vi "Set RX Output Divider.vi"(8 "error in":errorcluster, 10 "rx output divider":T1, 11 "eye scan in":refnum<class "niHighSpeedSerial Eye Scan v1 Host.lvclass">) -> (0 "error out":errorcluster, 3 "eye scan out":refnum<class "niHighSpeedSerial Eye Scan v1 Host.lvclass">)   [LabVIEW 2014, in "niHighSpeedSerial Eye Scan v1 Host.lvclass"]
doc: "Sets the RX Output Divider. This must match the values configured with RXRATE and RXOUT_DIV.\n\n<B>Input Parameters</B>\n\n<B>error in</B> describes error conditions that occur before this node runs. This input provides standard 'error in' functionality.\n\n<B>rx output divider</B> represents the configuration of the receiver output divider. This should match the values configured with RXRATE and RXOUT_DIV.\nenum values: 1,2,4,8,16\n\n<B>eye scan in</B> Takes in a reference to your session from the previous VI.\n\n<B>Output Parameters</B>\n\n<B>error out</B> contains error information. This output provides standard 'error out' functionality.\n\n<B>eye scan out</B> passes a reference to your session to the next VI."
uses:
  <instrlib>/niHighSpeedSerial/Eye Scan/v1/Host/Eye Scan/niHighSpeedSerial Eye Scan v1 Host.lvclass
  <instrlib>/niHighSpeedSerial/Eye Scan/v1/Host/Common/Public/RX Output Divider.ctl
  <instrlib>/niHighSpeedSerial/Eye Scan/v1/Host/Eye Scan/niHighSpeedSerial Eye Scan v1 Host.lvclass/niHighSpeedSerial Eye Scan v1 Host.ctl
  <vilib>/Utility/error.llb/Error Cluster From Error Code.vi
  <vilib>/ErrorRing/Error Ring.xnode
  <instrlib>/niHighSpeedSerial/Eye Scan/v1/Host/Common/niHighSpeedSerial Eye Scan Common v1 Host.lvlib
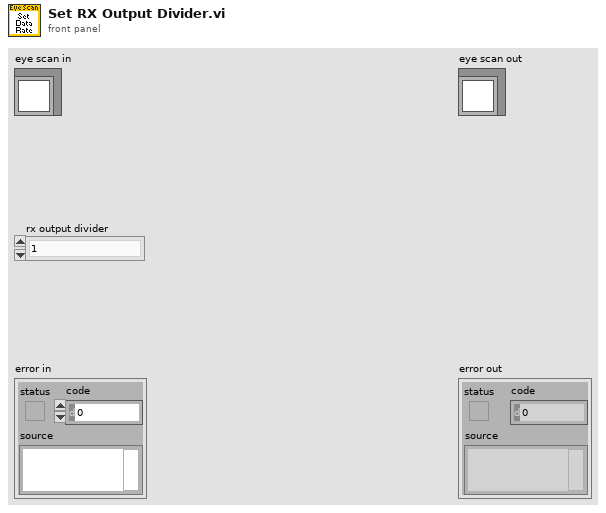
[diagram p1: front panel]
types:
  T1 = typedef "niHighSpeedSerial Eye Scan Common v1 Host.lvlib/RX Output Divider.ctl" = enum16{"1", "2", "4", "8", "16"}
  T2 = typedef "niHighSpeedSerial Eye Scan v1 Host.lvclass/Private Data.ctl" = cluster{"instruction target":refnum<class "niInstr Instruction Target v1 Host.lvclass">, "channels":T3[], "measure state":T4, "rx output divider":T1, "equalization mode":T5, "rx data width":T6, "BER floor":dbl, "number of points completed":i32, "rx output divider configured?":bool, "equalization mode configured?":bool, "rx data width configured?":bool}
  T3 = typedef "niHighSpeedSerial Eye Scan v1 Host.lvclass/Channel Data.ctl" = cluster{"instance":u8, "channel":refnum<class "niHighSpeedSerial Eye Scan Single Point v1 Host.lvclass">, "point iterator":refnum<class "niHighSpeedSerial Eye Scan Point Iterator v1 Host.lvclass">}
  T4 = typedef "niHighSpeedSerial Eye Scan v1 Host.lvclass/Measure State.ctl" = enum16{"Uninitialized", "Initialized", "Ready", "Measuring", "Finished", "Aborted"}
  T5 = typedef "niHighSpeedSerial Eye Scan Common v1 Host.lvlib/Equalization Mode.ctl" = enum16{"DFE", "LPM"}
  T6 = typedef "niHighSpeedSerial Eye Scan Common v1 Host.lvlib/Data Width.ctl" = enum16{"16 Bit", "20 Bit", "32 Bit", "40 Bit"}
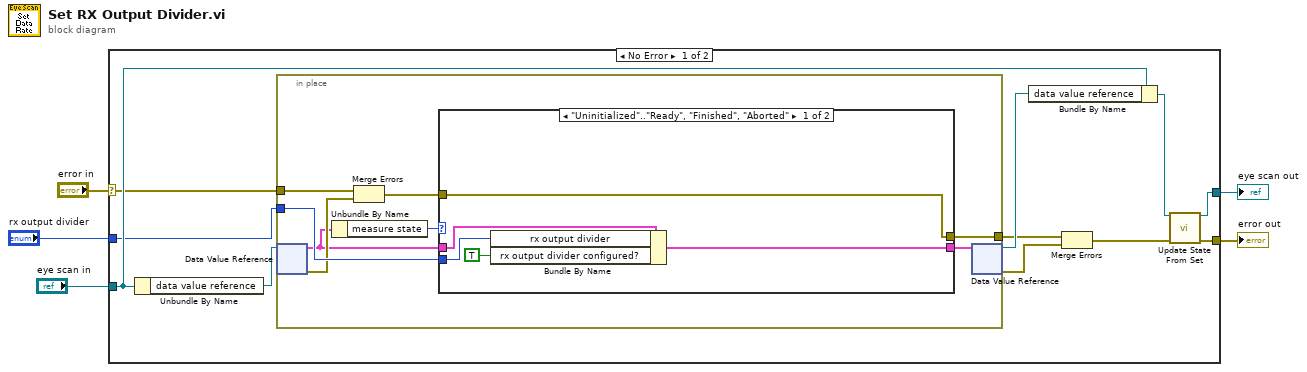
[diagram p0: block diagram]
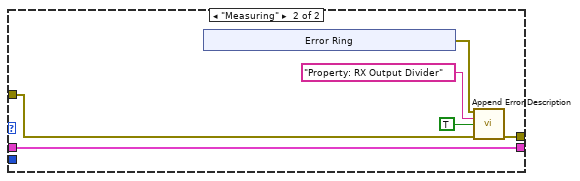
[diagram p2: hidden frame]
diagram:
  n1 = case shown="No Error" "error in" {
    selector: "error in" -> [w10 w41]
    tunnel: [w6 w41] -> w4
    tunnel: [w8 w40] -> w2
    tunnel: "eye scan in" -> [w14 w40]
    tunnel: "rx output divider" -> [w13 _]
    frame No Error {
      n2 = Unbundle By Name(w14) -> ("data value reference"=w16:refnum<data-value>)
      n3 = in-place {
        in-place-border: w13 -> [w24]
        in-place-border: [w19] -> w12
        in-place-border: w10 -> [w23]
        n4 = in-place-dvr #1(w16) -> (w17:T2, w22:errorcluster)
        n5 = Unbundle By Name(w17) -> ("measure state"=w20:T4)
        n6 = Merge Errors(w23, w22) -> (w21:errorcluster)
        n7 = case shown="\"Uninitialized\"..\"Ready\", \"Finished\", \"Aborted\"" w20 {
          tunnel: w21 -> [w29 w31]
          tunnel: [w29 w30] -> w19
          tunnel: w24 -> [w27 _]
          tunnel: w17 -> [w28 w35]
          tunnel: [w26 w35] -> w18
          frame "Uninitialized".."Ready", "Finished", "Aborted" {
            n8 = Bundle By Name(cluster=w28, "rx output divider"=w27, "rx output divider configured?"=TRUE) -> (w26:T2)
          }
          frame "Measuring" {
            n9 = xnode "Error Ring"() -> ("error out"=w34:errorcluster)
            n10 = call <instrlib>:"Append Error Description.vi"("error to append"=w34, "append string (\"\")"="Property: RX Output Divider" ("append string (\"\")"), "generate error?"=TRUE, "error in"=w31) -> ("error out"=w30:errorcluster)  [unwired: 11 in]
          }
        }
        n11 = in-place-dvr #1(w18) -> (w15:refnum<data-value>, w11:errorcluster)
      }
      n12 = Bundle By Name(cluster=w14, "data value reference"=w15) -> (w9:refnum<class "niHighSpeedSerial Eye Scan v1 Host.lvclass">)
      n13 = Merge Errors(w12, w11) -> (w7:errorcluster)
      n14 = call <instrlib>:"Update State From Set.vi"("eye scan in"=w9, "error in"=w7) -> ("eye scan out"=w8:refnum<class "niHighSpeedSerial Eye Scan v1 Host.lvclass">, "error out"=w6:errorcluster)  [unwired: 12 in]
    }
    frame Error {
    }
  }
  "error out" <- w4
  "eye scan out" <- w2
